vi "Server.vi"() -> ()   [LabVIEW 2015]
panel:
  in  "stop":bool
  out "data out":string
  out "error out":errorcluster
  in  "error in (no error)":errorcluster
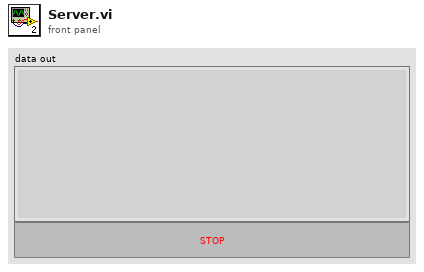
[diagram p1: front panel]
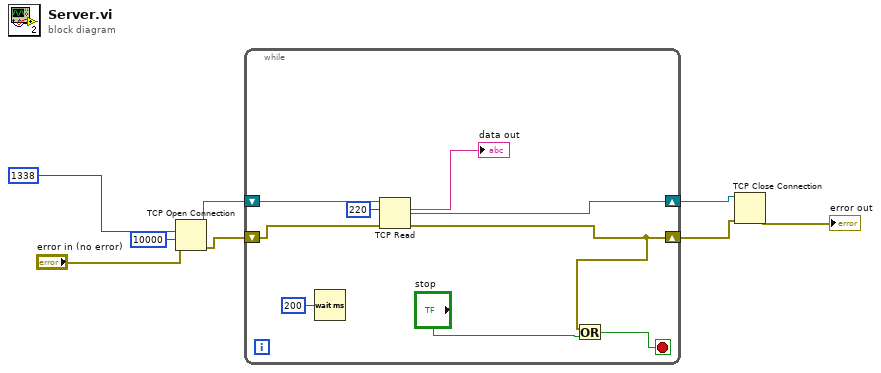
[diagram p0: block diagram]
diagram:
  n1 = TCP Open Connection(remote port or service name=u16 1338, timeout ms (60000)=10000, error in (no error)="error in (no error)") -> (connection ID=w7:refnum<k5>, error out=w1:errorcluster)  [unwired: 2 in]
  n2 = while {
    shift-right: [w11] -> w4
    shift-left: w7 -> [w17]
    shift-right: [w10] -> w3
    shift-left: w1 -> [w9]
    stop <- w13 stop-if-true
    n3 = Wait (ms)(milliseconds to wait=u32 200) -> ()  [unwired: 1 out]
    n4 = TCP Read(connection ID=w17, bytes to read=220, error in (no error)=w9) -> (connection ID out=w11:refnum<k5>, data out=→"data out":string, error out=w10:errorcluster)  [unwired: 2 in]
    n5 = Or(x=w10, y="stop") -> (x .or. y?=w13:bool)
  }
  n6 = TCP Close Connection(connection ID=w4, error in (no error)=w3) -> (error out=→"error out":errorcluster)  [unwired: 1 in, 1 out]
